vi "CONEX-ALL Get Positioner Error And Controller State v2.vi"(11 "Connection Cluster in":T1) -> (1 "Controller state":string, 2 "Positioner error":string, 3 "Connection Cluster out":T1)   [LabVIEW 2013]
doc: "TS? - Get Positioner Error and Controller State\n\nReturn:\n\nPositioner error portion of status code\nController status portion status code"
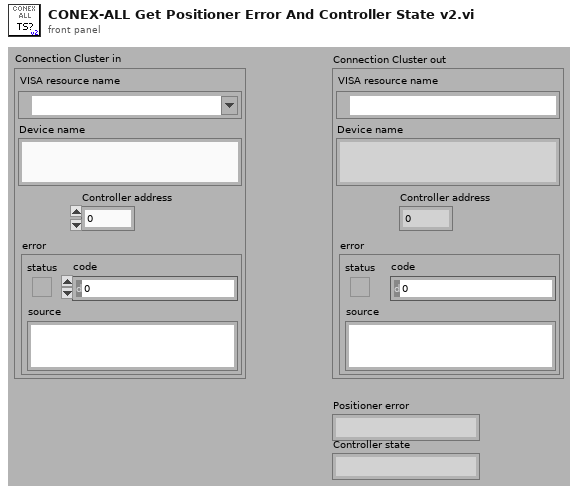
[diagram p1: front panel]
types:
  T1 = cluster{"VISA resource name":refnum<visa-resource-name>, "Device name":string, "Controller address":i32, "error":errorcluster}
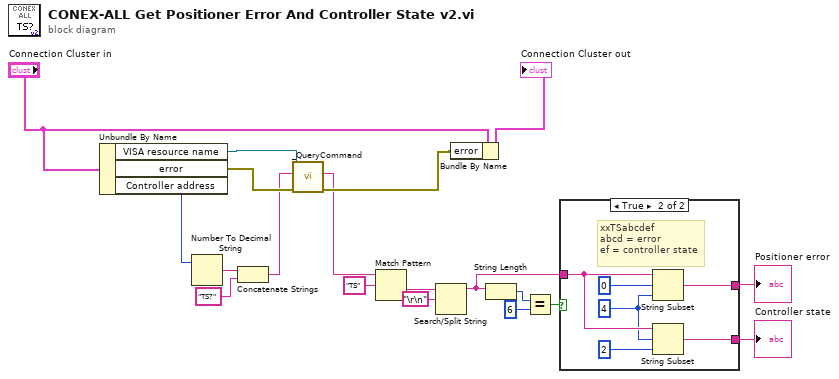
[diagram p0: block diagram]
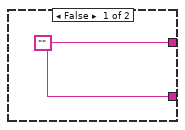
[diagram p2: hidden frame]
diagram:
  n1 = Unbundle By Name("Connection Cluster in") -> ("VISA resource name"=w8:refnum<visa-resource-name>, "error"=w6:errorcluster, "Controller address"=w3:i32)
  n2 = Number To Decimal String(number=w3) -> (decimal integer string=w19:string)  [unwired: 1 out]
  n3 = Concatenate Strings(w19, "TS?" ("strCommand")) -> (w2:string)
  n4 = call "_QueryCommand.vi"("error in"=w6, "Command"=w2, "Instrument Channel in"=w8) -> ("error out"=w7:errorcluster, "Response"=w1:string)  [unwired: 6 in, 1 out]
  n5 = Match Pattern(string=w1, regular expression="TS" ("expression régulière")) -> (after substring=w10:string)  [unwired: 4 out]
  n6 = Search/Split String(string=w10, search string/char (-)="\r\n") -> (substring before match=w9:string)  [unwired: 3 out]
  n7 = Bundle By Name(cluster="Connection Cluster in", "error"=w7) -> (→"Connection Cluster out":T1)
  n8 = String Length(string=w9) -> (length=w14:i32)
  n9 = Equal?(x=w14, y=6) -> (x = y?=w12:bool)
  n10 = case shown="True" w12 {
    tunnel: [w20 w25] -> w16
    tunnel: [w20 w21] -> w15
    tunnel: w9 -> [_ w24]
    frame False {
      w20 = ""
    }
    frame True {
      w22 = 4 ("longueur (reste)")
      # "xxTSabcdef\nabcd = error\nef = controller state"
      n11 = String Subset(string=w24, offset (0)=0, length (rest)=w22) -> (substring=w25:string)
      n12 = String Subset(string=w24, offset (0)=w22, length (rest)=2 ("longueur (reste)")) -> (substring=w21:string)
    }
  }
  "Positioner error" <- w16
  "Controller state" <- w15
